vi "Pump Manual Commands.vi"(7 "Write (F)":bool, 10 "Pumps Enabled IN":bool[](array[boolean]), 11 "Manual CMDs IN":dbl[](array[numeric])) -> (2 "Pumps Enabled OUT":bool[](array[boolean]), 3 "Manual CMDs OUT":dbl[](array[numeric]))   [LabVIEW 2019]
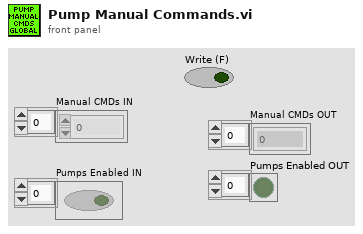
[diagram p1: front panel]
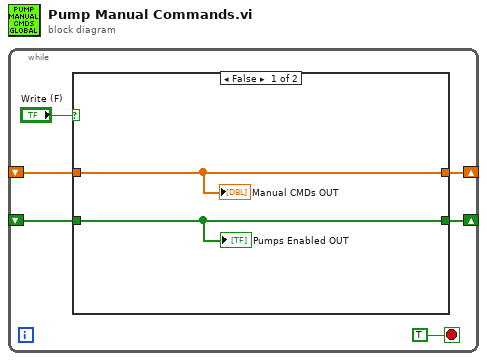
[diagram p0: block diagram]
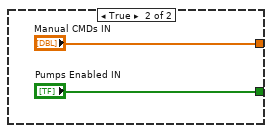
[diagram p2: hidden frame]
diagram:
  n1 = while {
    shift-right: [w4] -> _
    shift-left: _ -> [w2]
    shift-right: [w3] -> _
    shift-left: _ -> [w1]
    stop <- TRUE stop-if-true
    n2 = case shown="False" "Write (F)" {
      tunnel: [w8 "Manual CMDs IN"] -> w4
      tunnel: [w7 "Pumps Enabled IN"] -> w3
      tunnel: w2 -> [w8 _]
      tunnel: w1 -> [w7 _]
      frame False {
        "Manual CMDs OUT" <- w8
        "Pumps Enabled OUT" <- w7
      }
      frame True {
      }
    }
  }
